vi "test_Export Configuration_Group.vi"(8 "error in (no error)":errorcluster, 11 "TestCase in":refnum<class "FPGA Addon Scripting API Unit Tests.lvclass">) -> (0 "error out":errorcluster, 3 "TestCase out":refnum<class "FPGA Addon Scripting API Unit Tests.lvclass">)   [LabVIEW 2021, in "FPGA Addon Scripting API Unit Tests.lvclass"]
uses:
  FPGA Addon Scripting API Unit Tests.lvclass
  APIs/Scripting API/TypeDefs/Input Scalar Data.ctl
  APIs/Scripting API/Public/Bitfile Resources/Import Bitfile Scalars (Instances)/Import Scalars - by label.vi
  <vilib>/addons/_JKI Toolkits/VI Tester/TestCase.llb/TestCase.lvclass
  FPGA Addon Test Class/FPGA Addon Test Class.lvclass
  APIs/Scripting API/Scripting API.lvlib
  C:/Program Files/National Instruments/LabVIEW 2021/vi.lib/addons/_JKI Toolkits/VI Tester/TestCase.llb/TestCase.lvclass
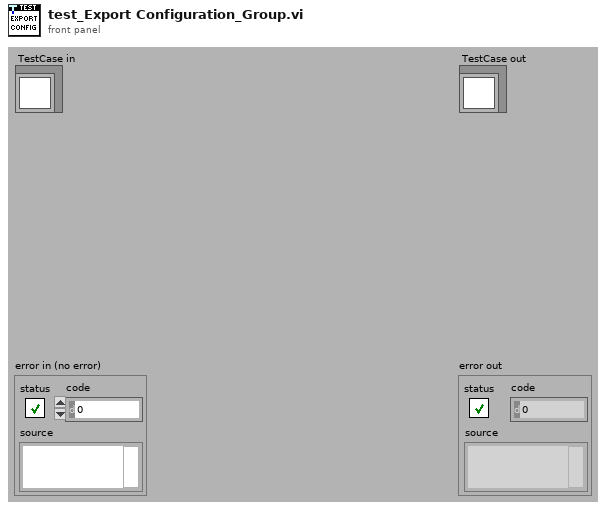
[diagram p1: front panel]
types:
  T1 = typedef "Scripting API.lvlib/Input Scalar Data.ctl" = cluster{"Bitfile Name":string, "SysDef Name":string}
  T2 = typedef "Custom Device API.lvlib/Custom Device Item Ref.ctl" = u64
  T3 = typedef "Scripting API.lvlib/Output Scalar Data.ctl" = cluster{"Bitfile Name":string, "SysDef Channel Name":string, "Imported":bool, "Data Type":T4}
  T4 = typedef "FPGA Addon Shared.lvlib/FPGA Addon Data Type.ctl" = enum8{"<Null>", "I8", "I16", "I32", "I64", "U8", "U16", "U32", "U64", "SGL", "Boolean", "Analog PWM In Settings", "Analog PWM In", "Digital PWM In Settings", "Digital PWM In", "Digital PWM Out", "Sine Out", "FXP", "FXP+/-24.5", "FXP+/-16.5", "FXP+/-32.8", "FXP+/-64.32", "FXP+/-16.7", "FXP+/-20.5", "FXP+/-27.5", "FXP+/-32.16", "FXP+16.3", "FXP+18.3", "Digital Static In", "Digital Static Out", "Digital Static In Settings", "Digital WSS Out", "Quad Encoder Settings", "Quad Encoder In", "Group"}
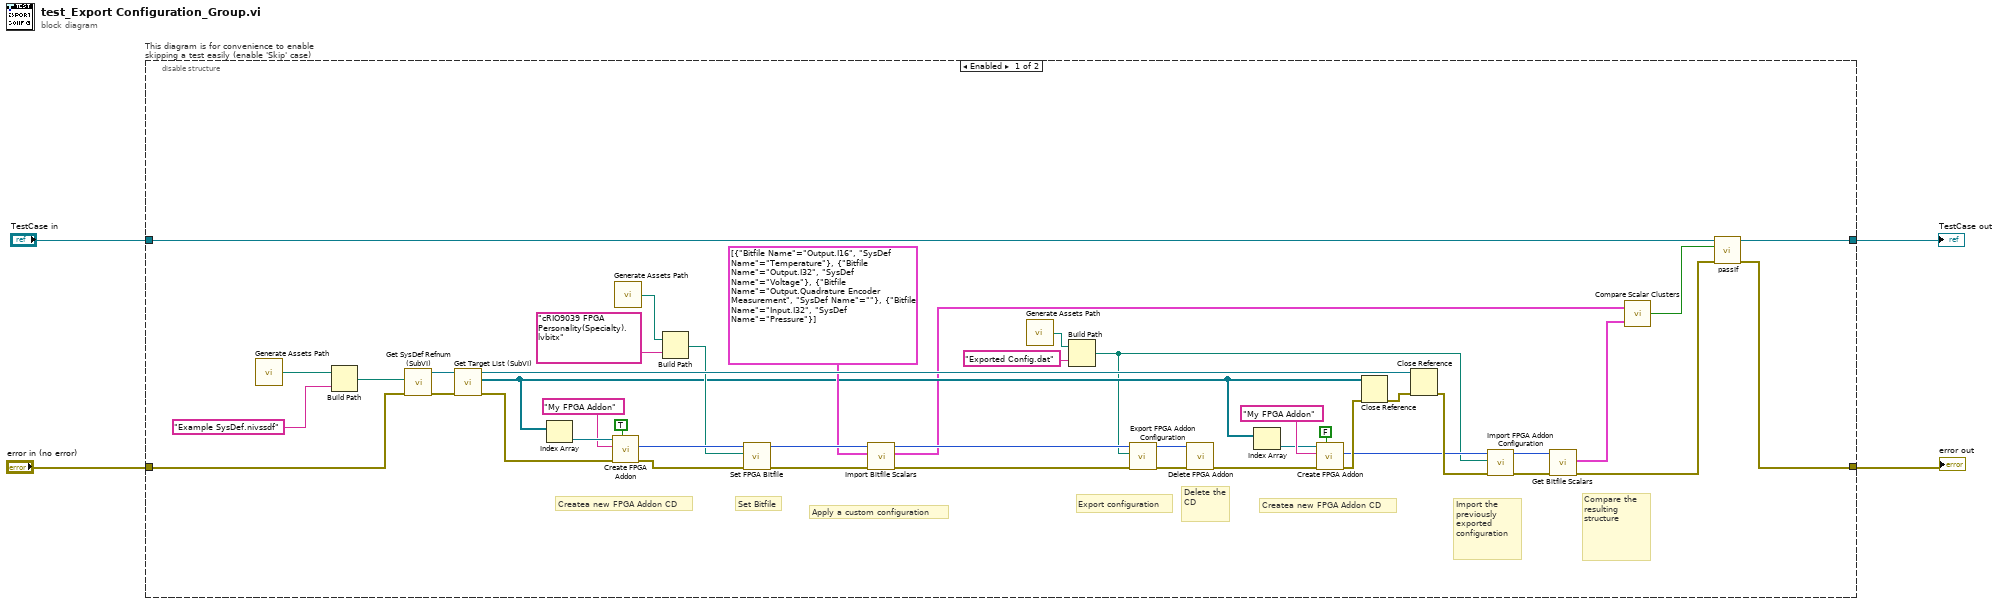
[diagram p0: block diagram]
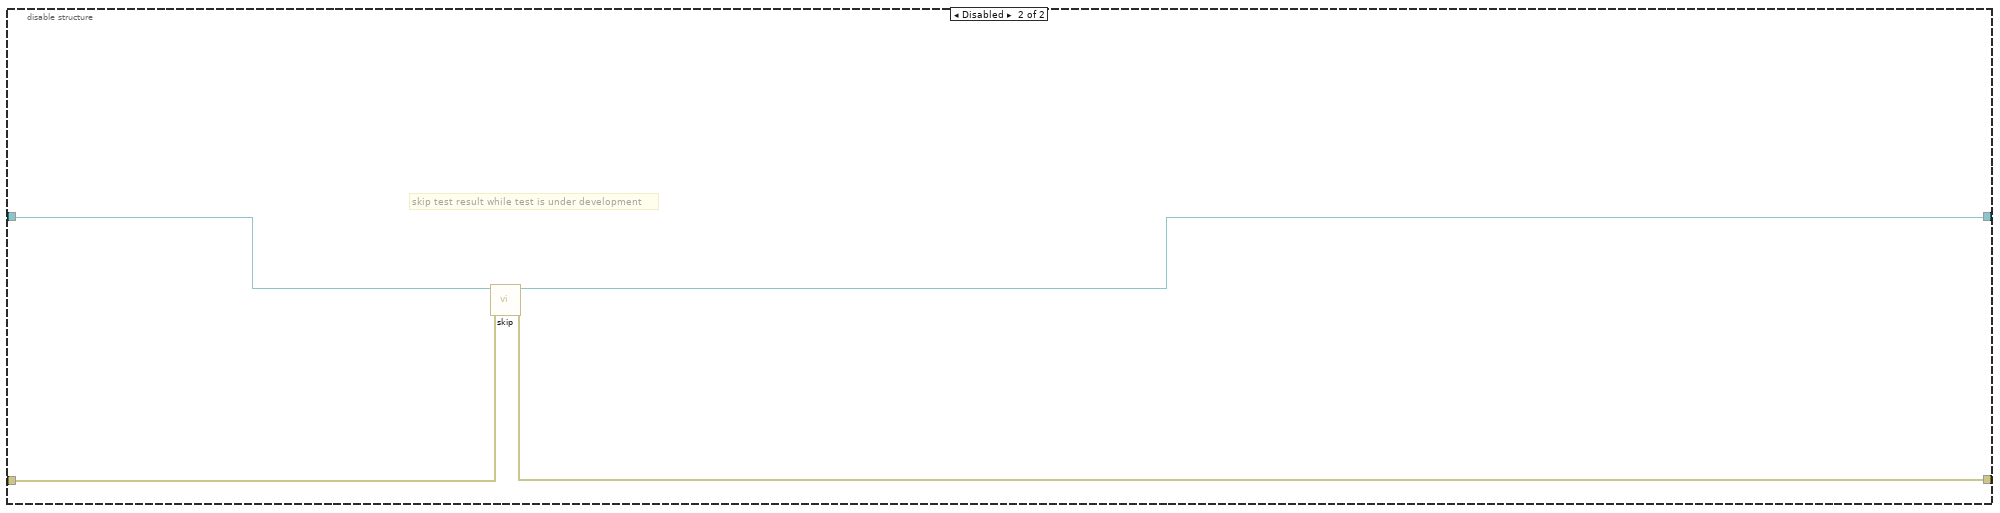
[diagram p2: hidden frame]
diagram:
  n1 = disable-structure "This diagram is for convenience to enable skipping a test easily (enable 'Skip' case)" shown="Enabled" {
    disable-tunnel: "TestCase in" -> [w9 w52]
    disable-tunnel: [w8 w50] -> w1
    disable-tunnel: [w5 w51] -> w3
    disable-tunnel: "error in (no error)" -> [w42 w49]
    frame Enabled {
      # "Compare the resulting structure"
      # "Import the previously exported configuration"
      # "Createa new FPGA Addon CD"
      # "Delete the CD"
      # "Export configuration"
      # "Apply a custom configuration"
      # "Set Bitfile"
      # "Createa new FPGA Addon CD"
      n2 = call "Generate Assets Path.vi"() -> ("Assets path"=w48:path)
      n3 = Build Path(base path=w48, name or relative path="Example SysDef.nivssdf") -> (appended path=w46:path)
      n4 = call "Get SysDef Refnum (SubVI).vi"("error in (no error)"=w42, "System Definition path"=w46) -> ("error out"=w41:errorcluster, "SysDef Refnum out"=w45:refnum<k24>)  [unwired: 8 in]
      n5 = call "Get Target List (SubVI).vi"("error in (no error)"=w41, "SysDef Refnum in"=w45) -> ("error out"=w40:errorcluster, "Target List Refnums"=w19:refnum<k24>[], "SysDef Refnum out"=w39:refnum<k24>)  [unwired: 7 in]
      n6 = Index Array(array=w19) -> (element=w44:refnum<k24>)  [unwired: 1 in]
      n7 = call "Create FPGA Addon.vi"("group scalars"=TRUE, "error in"=w40, "FPGA addon name"="My FPGA Addon", "target in"=w44) -> ("error out"=w23:errorcluster, "FPGA addon refnum"=w36:T2)  [unwired: 5 in, 1 out]
      n8 = call "Generate Assets Path.vi"() -> ("Assets path"=w35:path)
      n9 = Build Path(base path=w35, name or relative path="cRIO9039 FPGA Personality(Specialty).lvbitx") -> (appended path=w33:path)
      n10 = call "Set FPGA Bitfile.vi"("error in"=w23, "FPGA bitfile path"=w33, "FPGA addon refnum in"=w36) -> ("error out"=w32:errorcluster, "FPGA addon refnum out"=w31:T2)  [unwired: 7 in]
      n11 = call-poly "Import Bitfile Scalars.vi"("error in"=w32, "bitfile scalars in"=T1[] [{"Bitfile Name"="Output.I16", "SysDef Name"="Temperature"}, {"Bitfile Name"="Output.I32", "SysDef Name"="Voltage"}, {"Bitfile Name"="Output.Quadrature Encoder Measurement", "SysDef Name"=""}, {"Bitfile Name"="Input.I32", "SysDef Name"="Pressure"}], "FPGA addon refnum in"=w31) -> ("error out"=w29:errorcluster, "imported bitfile scalars out"=w10:T3[], "FPGA addon refnum out"=w28:T2)  [unwired: 6 in]
      n12 = call "Generate Assets Path.vi"() -> ("Assets path"=w27:path)
      n13 = Build Path(base path=w27, name or relative path="Exported Config.dat") -> (appended path=w14:path)
      n14 = call "Export FPGA Addon Configuration.vi"("error in"=w29, "export file path"=w14, "FPGA addon refnum in"=w28) -> ("error out"=w25:errorcluster, "FPGA addon refnum out"=w24:T2)  [unwired: 7 in]
      n15 = call "Delete FPGA Addon.vi"("error in"=w25, "FPGA addon refnum"=w24) -> ("error out"=w20:errorcluster)  [unwired: 8 in, 1 out]
      n16 = Index Array(array=w19) -> (element=w18:refnum<k24>)  [unwired: 1 in]
      n17 = call "Create FPGA Addon.vi"("group scalars"=FALSE, "error in"=w20, "FPGA addon name"="My FPGA Addon", "target in"=w18) -> ("error out"=w17:errorcluster, "FPGA addon refnum"=w15:T2)  [unwired: 5 in, 1 out]
      n18 = Close Reference(reference=w19, error in (no error)=w17) -> (error out=w38:errorcluster)
      n19 = Close Reference(reference=w39, error in (no error)=w38) -> (error out=w16:errorcluster)
      n20 = call "Import FPGA Addon Configuration.vi"("error in"=w16, "configuration file path"=w14, "FPGA addon refnum in"=w15) -> ("error out"=w13:errorcluster, "FPGA addon refnum out"=w12:T2)  [unwired: 7 in]
      n21 = call "Get Bitfile Scalars.vi"("error in"=w13, "FPGA addon refnum in"=w12) -> ("error out"=w6:errorcluster, "bitfile scalars out"=w11:T3[])  [unwired: 7 in, 1 out]
      n22 = call "Compare Scalar Clusters.vi"("Target bitfile scalars in"=w11, "Reference bitfile scalars in"=w10) -> ("Equal ?"=w7:bool)
      n23 = call-dynamic "passIf.vi"("error in (no error)"=w6, "pass"=w7, "TestCase in"=w9) -> ("error out"=w5:errorcluster, "TestCase out"=w8:refnum<class "FPGA Addon Scripting API Unit Tests.lvclass">)  [unwired: 7 in]
    }
    frame Disabled {
      # "skip test result while test is under development"
      n24 = call <vilib>:"skip.vi"("error in (no error)"=w49, "TestCase in"=w52) -> ("error out"=w51:errorcluster, "TestCase out"=w50:refnum<class "FPGA Addon Scripting API Unit Tests.lvclass">)  [unwired: 8 in]
    }
  }
  "error out" <- w3
  "TestCase out" <- w1
